vi "MainV2.vi"() -> ()   [LabVIEW 2015]
uses:
  <vilib>/MakerHub/LINX/Public/Peripherals/Digital/Digital Write N Chans.vi
  <vilib>/MakerHub/LINX/Public/Peripherals/Digital/Digital Write 1 Chan.vi
  <vilib>/MakerHub/LINX/Public/Peripherals/Digital/Digital Read 1 Chan.vi
  <vilib>/MakerHub/LINX/Private/Local IO/LinxDigitalWrite.vi
  <vilib>/MakerHub/LINX/Public/Utilities/Check Channel.vi
  <vilib>/MakerHub/LINX/Public/Peripherals/Digital/Digital Read N Chans.vi
  <vilib>/MakerHub/LINX/Private/Local IO/LinxDigitalRead.vi
  <vilib>/MakerHub/LINX/Public/Utilities/Open Serial.vi
  <vilib>/MakerHub/LINX/Private/Utilties/Generate Error.vi
  <vilib>/MakerHub/LINX/LMH-LINX.lvlib
panel:
  in  "Process Stop Button 2":bool
  out "Robot Source Code":string
  out "WorkPiece in Polishing Process":T1(plugin-control)
  out "Arduino Error Out":errorcluster
  out "Robot Polishing Status":bool
  in  "Play Button":bool
  in  "Process Stop Button":bool
  out "PROCESS STATE":T2(ring)
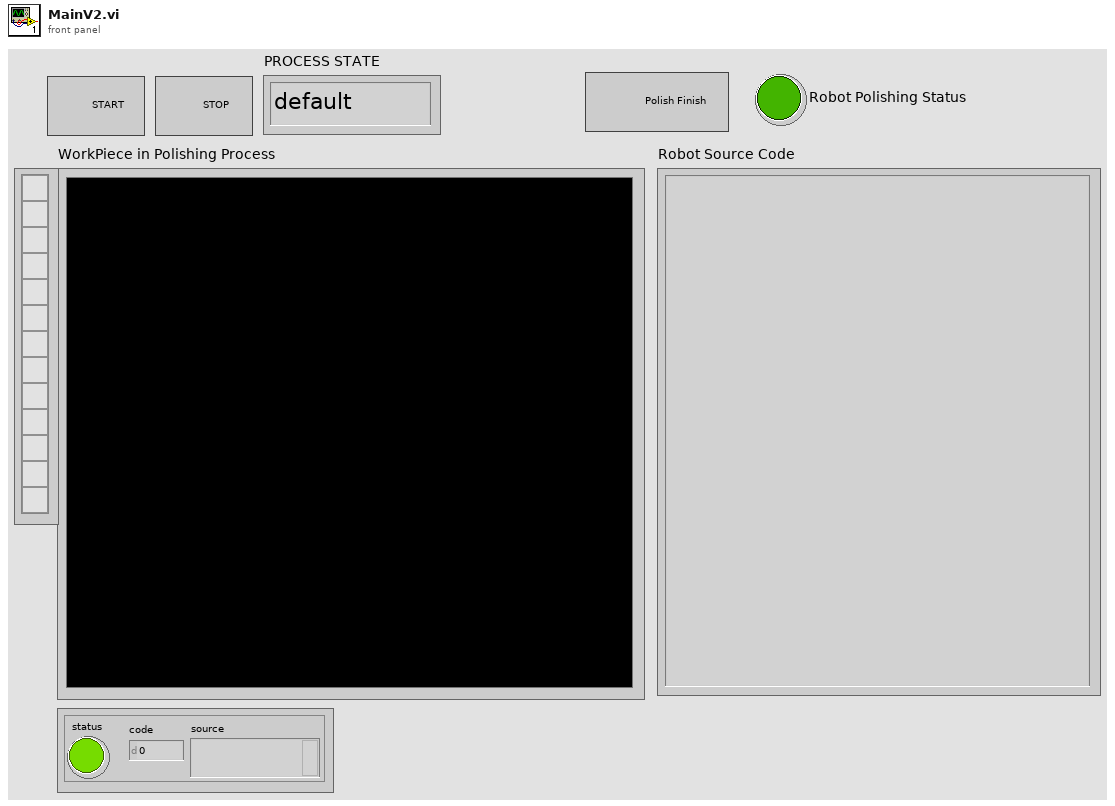
[diagram p1: front panel]
types:
  T1 = typedef "IMAQ Image.ctl" = refnum<image>
  T2 = enum16{"default", "Initial", "Conveyor", "Vision", "Polish", "ShiftJig", "Stop", ""}
  T3 = typedef "LMH-LINX.lvlib/LINX Ref.ctl" = cluster{"IO":T4, "Interface":T5, "LINX Device Config":T6}
  T4 = typedef "LMH-LINX.lvlib/Platform.ctl" = enum16{"Remote", "Local"}
  T5 = typedef "LMH-LINX.lvlib/Interface.ctl" = enum16{"Serial", "TCP"}
  T6 = typedef "LMH-LINX.lvlib/Device.lvlib/LINX Device Config.ctl" = cluster{"Interface":T5, "COM Port":refnum<visa-resource-name>, "TCP Configuration":T7, "Device Family":u8, "Device ID":u8, "Device Name":string, "TCP Ref":refnum<k5>, "Channels":T8}
  T7 = typedef "LMH-LINX.lvlib/Device.lvlib/TCP Config.ctl" = cluster{"IP Address":string, "Port":u16}
  T8 = typedef "LMH-LINX.lvlib/Channels.ctl" = cluster{"DI":u8[], "DO":u8[], "AI":u8[], "AO":u8[], "PWM":u8[], "QE":u8[], "UART":u8[], "I2C 2":u8[], "SPI":u8[], "CAN":u8[], "Servo":u8[], "AI Ref (V)":dbl, "AI Resolution (Bits)":u8, "AO Ref (V)":dbl, "AO Resolution (Bits)":u8}
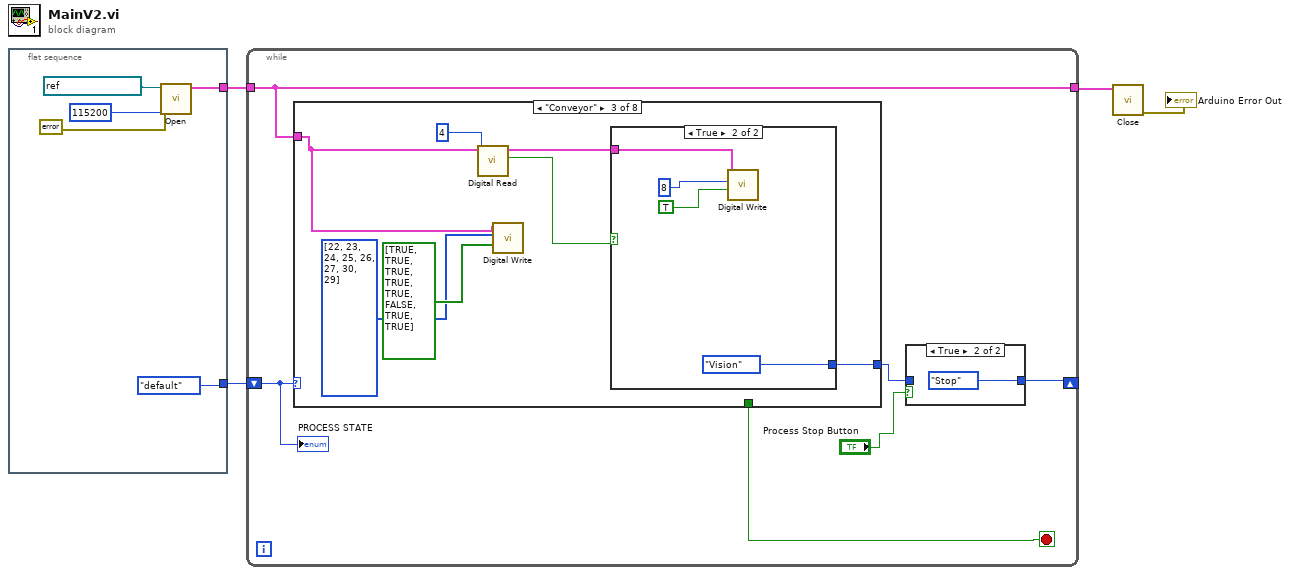
[diagram p0: block diagram]
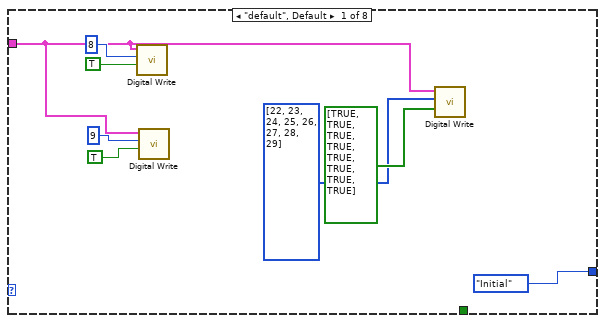
[diagram p3: hidden frame]
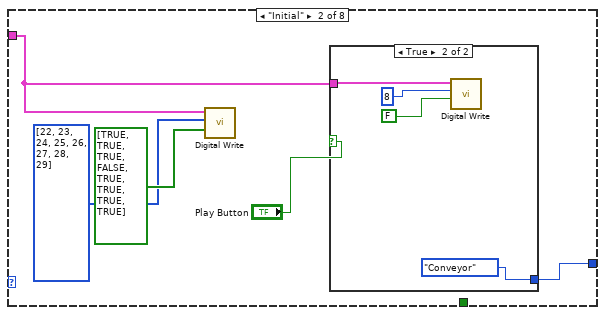
[diagram p4: hidden frame]
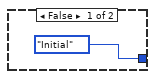
[diagram p5: hidden frame]
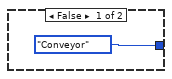
[diagram p6: hidden frame]
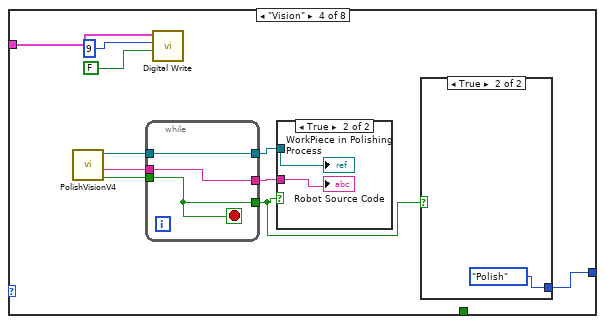
[diagram p7: hidden frame]
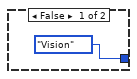
[diagram p9: hidden frame]
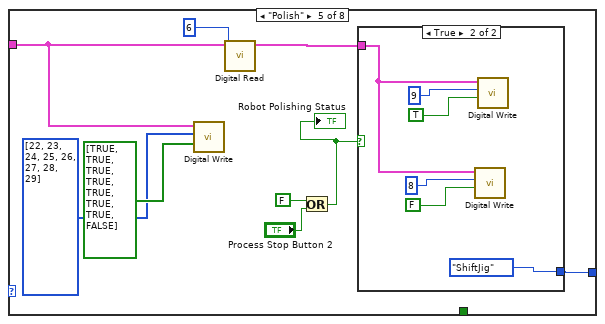
[diagram p10: hidden frame]
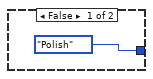
[diagram p11: hidden frame]
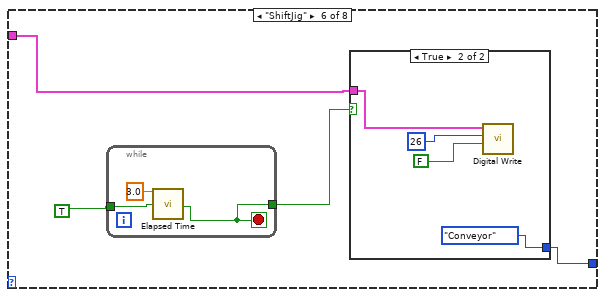
[diagram p12: hidden frame]
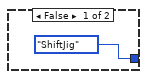
[diagram p13: hidden frame]
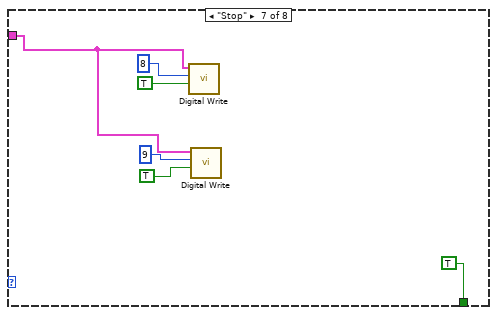
[diagram p14: hidden frame]
diagram:
  n1 = flat-sequence {
    tunnel: [T2."default"] -> w4
    tunnel: [w6] -> w3
    frame #0 {
      n2 = call-poly <vilib>:"Open.vi"("Error In"=errorcluster {"status"=FALSE, "code"=0, "source"=""}, "Baud Rate Override"=u32 115200, "Serial Port"=refnum<visa-resource-name> "COM4") -> ("LINX Resource"=w6:T3)  [unwired: 6 in, 2 out]
    }
  }
  n3 = while {
    tunnel: w3 -> [w14]
    shift-right: [w12] -> _
    shift-left: w4 -> [w15]
    tunnel: [w14] -> w1
    stop <- w10 stop-if-true
    n4 = case shown="\"Conveyor\"" w15 {
      tunnel: w14 -> [w19 w26 w36 w55 w66 w81 w94 _]
      tunnel: [T2."Initial" w29 w41 w54 w71 w84 _ _] -> w11
      tunnel: [_ _ _ _ _ _ TRUE _] -> w10
      frame "default", Default {
        n5 = call-poly <vilib>:"Digital Write.vi"("Output Value"=TRUE, "DO Channel"=u8 8, "LINX Resource"=w19) -> ()  [unwired: 7 in, 2 out]
        n6 = call-poly <vilib>:"Digital Write.vi"("Output Value"=TRUE, "DO Channel"=u8 9, "LINX Resource"=w19) -> ()  [unwired: 7 in, 2 out]
        n7 = call-poly <vilib>:"Digital Write.vi"("Values"=bool[] [TRUE, TRUE, TRUE, TRUE, TRUE, TRUE, TRUE, TRUE], "DO Channels"=u8[] [22, 23, 24, 25, 26, 27, 28, 29], "LINX Resource"=w19) -> ()  [unwired: 7 in, 2 out]
      }
      frame "Initial" {
        n8 = call-poly <vilib>:"Digital Write.vi"("Values"=bool[] [TRUE, TRUE, TRUE, FALSE, TRUE, TRUE, TRUE, TRUE], "DO Channels"=u8[] [22, 23, 24, 25, 26, 27, 28, 29], "LINX Resource"=w26) -> ()  [unwired: 7 in, 2 out]
        n9 = case shown="True" "Play Button" {
          tunnel: [T2."Initial" T2."Conveyor"] -> w29
          tunnel: w26 -> [_ w32]
          frame False {
          }
          frame True {
            n10 = call-poly <vilib>:"Digital Write.vi"("Output Value"=FALSE, "DO Channel"=u8 8, "LINX Resource"=w32) -> ()  [unwired: 7 in, 2 out]
          }
        }
      }
      frame "Conveyor" {
        n11 = call-poly <vilib>:"Digital Read.vi"("DI Channel"=u8 4, "LINX Resource"=w36) -> ("DI Value"=w39:bool, "LINX Resource"=w40:T3)  [unwired: 7 in, 1 out]
        n12 = call-poly <vilib>:"Digital Write.vi"("Values"=bool[] [TRUE, TRUE, TRUE, TRUE, TRUE, FALSE, TRUE, TRUE], "DO Channels"=u8[] [22, 23, 24, 25, 26, 27, 30, 29], "LINX Resource"=w36) -> ()  [unwired: 7 in, 2 out]
        n13 = case shown="True" w39 {
          tunnel: [T2."Conveyor" T2."Vision"] -> w41
          tunnel: w40 -> [_ w44]
          frame False {
          }
          frame True {
            n14 = call-poly <vilib>:"Digital Write.vi"("Output Value"=TRUE, "DO Channel"=u8 8, "LINX Resource"=w44) -> ()  [unwired: 7 in, 2 out]
          }
        }
      }
      frame "Vision" {
        n15 = call "PolishVisionV4.vi"() -> ("Status"=w52:bool, "Source CODE Robot"=w51:string, "WorkPiece In Process"=w53:T1)  [unwired: 9 in]
        n16 = while {
          tunnel: w53 -> [w62]
          tunnel: [w62] -> w50
          tunnel: w52 -> [w60]
          tunnel: w51 -> [w61]
          tunnel: [w61] -> w49
          tunnel: [w60] -> w48
          stop <- w60 stop-if-true
        }
        n17 = call-poly <vilib>:"Digital Write.vi"("Output Value"=FALSE, "DO Channel"=u8 9, "LINX Resource"=w55) -> ()  [unwired: 7 in, 2 out]
        n18 = case shown="True" w48 {
          tunnel: w50 -> [_ w59]
          tunnel: w49 -> [_ w58]
          frame False {
          }
          frame True {
            "WorkPiece in Polishing Process" <- w59
            "Robot Source Code" <- w58
          }
        }
        n19 = case shown="True" w48 {
          tunnel: [T2."Vision" T2."Polish"] -> w54
          frame False {
          }
          frame True {
          }
        }
      }
      frame "Polish" {
        n20 = call-poly <vilib>:"Digital Write.vi"("Values"=bool[] [TRUE, TRUE, TRUE, TRUE, TRUE, TRUE, TRUE, FALSE], "DO Channels"=u8[] [22, 23, 24, 25, 26, 27, 28, 29], "LINX Resource"=w66) -> ()  [unwired: 7 in, 2 out]
        n21 = call-poly <vilib>:"Digital Read.vi"("DI Channel"=u8 6, "LINX Resource"=w66) -> ("LINX Resource"=w72:T3)  [unwired: 7 in, 2 out]
        n22 = Or(x=FALSE, y="Process Stop Button 2") -> (x .or. y?=w69:bool)
        "Robot Polishing Status" <- w69
        n23 = case shown="True" w69 {
          tunnel: [T2."Polish" T2."ShiftJig"] -> w71
          tunnel: w72 -> [_ w75]
          frame False {
          }
          frame True {
            n24 = call-poly <vilib>:"Digital Write.vi"("Output Value"=FALSE, "DO Channel"=u8 8, "LINX Resource"=w75) -> ()  [unwired: 7 in, 2 out]
            n25 = call-poly <vilib>:"Digital Write.vi"("Output Value"=TRUE, "DO Channel"=u8 9, "LINX Resource"=w75) -> ()  [unwired: 7 in, 2 out]
          }
        }
      }
      frame "ShiftJig" {
        n26 = while {
          tunnel: TRUE ("Auto Reset") -> [w86]
          tunnel: [w85] -> w82
          stop <- w85 stop-if-true
          n27 = call "Elapsed Time"("Time Target (s)"=3.0, "Auto Reset"=w86) -> ("Time has Elapsed"=w85:bool)  [unwired: 10 in, 7 out]
        }
        n28 = case shown="True" w82 {
          tunnel: [T2."ShiftJig" T2."Conveyor"] -> w84
          tunnel: w81 -> [_ w89]
          frame False {
          }
          frame True {
            n29 = call-poly <vilib>:"Digital Write.vi"("Output Value"=FALSE, "DO Channel"=u8 26, "LINX Resource"=w89) -> ()  [unwired: 7 in, 2 out]
          }
        }
      }
      frame "Stop" {
        n30 = call-poly <vilib>:"Digital Write.vi"("Output Value"=TRUE, "DO Channel"=u8 8, "LINX Resource"=w94) -> ()  [unwired: 7 in, 2 out]
        n31 = call-poly <vilib>:"Digital Write.vi"("Output Value"=TRUE, "DO Channel"=u8 9, "LINX Resource"=w94) -> ()  [unwired: 7 in, 2 out]
      }
      frame "" {
      }
    }
    n32 = case shown="True" "Process Stop Button" {
      tunnel: [w16 T2."Stop"] -> w12
      tunnel: w11 -> [w16 _]
      frame False {
      }
      frame True {
      }
    }
    "PROCESS STATE" <- w15
  }
  n33 = call <vilib>:"Close.vi"("LINX Resource"=w1) -> ("Error Out"=→"Arduino Error Out":errorcluster)  [unwired: 10 in]
